vi "Rigid Connection Command Filter.vi"(7 "Rigid Connection":bool, 10 "LBCB 2 Commands In":dbl[](array[numeric]), 11 "LBCB 1 Commands In":dbl[](array[numeric])) -> (2 "LBCB 2 Commands Out":dbl[](array[numeric]), 3 "LBCB 1 Commands Out":dbl[](array[numeric]))   [LabVIEW 2009]
uses:
  Data Access Objects/Metadata/DAO Actions.ctl
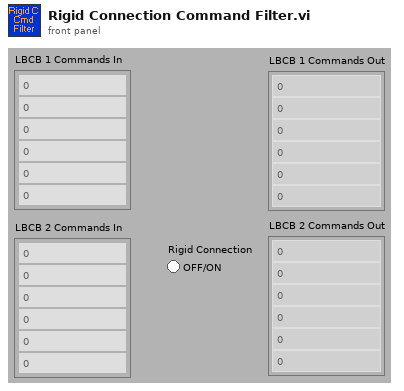
[diagram p1: front panel]
types:
  T1 = typedef "DAO Actions.ctl" = enum16{"Init", "Get", "Set"}
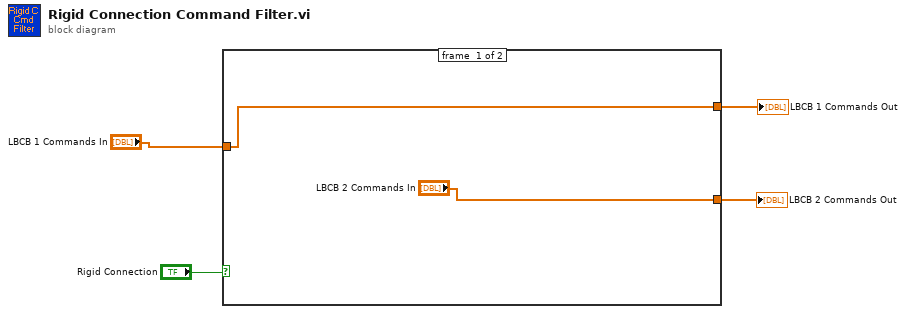
[diagram p0: block diagram]
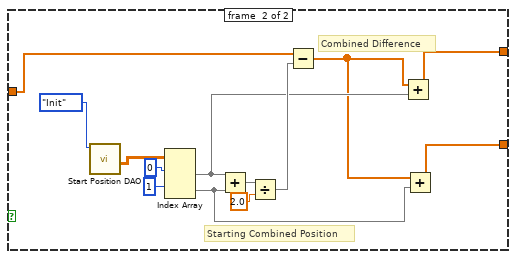
[diagram p2: hidden frame]
diagram:
  n1 = case shown="True" "Rigid Connection" {
    tunnel: [w5 w7] -> w3
    tunnel: ["LBCB 2 Commands In" w9] -> w1
    tunnel: "LBCB 1 Commands In" -> [w5 w8]
    frame #0 {
    }
    frame #1 {
      # "Combined Difference"
      # "Starting Combined Position"
      n2 = call "Start Position DAO.vi"("DAO Actions"=DAO_Actions."Init") -> ("Displacements Out"=w18:dbl[][])  [unwired: 9 in, 1 out]
      n3 = Index Array(array=w18, index (row) #1=0 ("index (row)"), index (row) #2=1 ("index (row)")) -> (element #1=w12:dbl[], element #2=w10:dbl[])  [unwired: 2 in]
      n4 = Add(x=w12, y=w10) -> (x+y=w13:dbl[])
      n5 = Divide(x=w13, y=2.0) -> (x/y=w14:dbl[])
      n6 = Subtract(x=w8, y=w14) -> (x-y=w11:dbl[])
      n7 = Add(x=w11, y=w12) -> (x+y=w7:dbl[])
      n8 = Add(x=w11, y=w10) -> (x+y=w9:dbl[])
    }
  }
  "LBCB 1 Commands Out" <- w3
  "LBCB 2 Commands Out" <- w1
